vi "Swerve Offset.vi"() -> ()   [LabVIEW 2017]
uses:
  Robot Global Data.vi
  <vilib>/Rock Robotics/WPI/ThirdParty/Phoenix-LabVIEW/Motor Controller/Get/CTRE_Phoenix_MotorController_GetPulseWidthAll.vi
panel:
  in  "Z":dbl(slide) scale=-1.0..1.0
  in  "X":dbl(slide) scale=-1.0..1.0
  in  "Y":dbl(slide)=0.2448979591836733 scale=-1.0..1.0
  in  "Offsets":dbl[](array[knob])=[-0.26448025674899267, -0.387138341978177, -0.11650266473879117, -0.12073098447218328] scale=-0.5..0.5
  in  "Change":bool
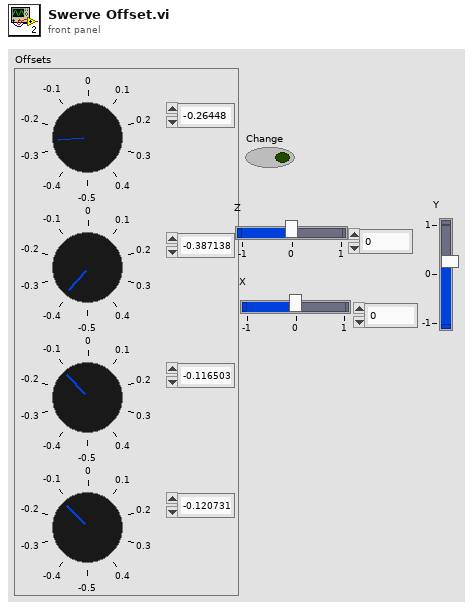
[diagram p1: front panel]
types:
  T1 = typedef "WPI_MotorControlDeviceRef.ctl" = cluster{"DeviceStatus":errorcluster, "Type":T2, "PWM":cluster{"PWM Channel":T3, "DeadBand":T4}, "CAN":cluster{"Device Number":u8, "SetOutput VI Ref":variant, "GetOutput VI Ref":variant, "Enable VI Ref":variant, "Disable VI Ref":variant, "Data":variant}, "Invert":bool, "DIO PWM":cluster{"PWM \"Enable\" Channel":T3, "DIOChannel":T5, "PWM Rate":dbl}}
  T2 = typedef "WPI_MotorControlType.ctl" = enum16{"PWM", "CAN", "DIO PWM"}
  T3 = typedef "FPGA_DIOPWMChannel.ctl" = enum8{"PWM 0", "PWM 1", "PWM 2", "PWM 3", "PWM 4", "PWM 5", "PWM 6", "PWM 7", "PWM 8", "PWM 9", "PWM MXP 0", "PWM MXP 1", "PWM MXP 2", "PWM MXP 3", "PWM MXP 4", "PWM MXP 5", "PWM MXP 6", "PWM MXP 7", "PWM MXP 8", "PWM MXP 9", "Invalid"}
  T4 = typedef "WPI_PWMDeadband.ctl" = cluster{"Name":string, "maxPositivePwm":i32, "minPositivePwm":i32, "centerPwm":i32, "maxNegativePwm":i32, "minNegativePwm":i32, "angularRange":u16}
  T5 = typedef "FPGA_DIOChannel.ctl" = enum8{"DIO 0", "DIO 1", "DIO 2", "DIO 3", "DIO 4", "DIO 5", "DIO 6", "DIO 7", "DIO 8", "DIO 9", "DIO MXP 0", "DIO MXP 1", "DIO MXP 2", "DIO MXP 3", "DIO MXP 4", "DIO MXP 5", "DIO MXP 6", "DIO MXP 7", "DIO MXP 8", "DIO MXP 9", "DIO MXP 10", "DIO MXP 11", "DIO MXP 12", "DIO MXP 13", "DIO MXP 14", "DIO MXP 15", "SPI Port CS1", "SPI Port CS2", "SPI Port CS3", "SPI Port MISO", "SPI Port MOSI", "Invalid"}
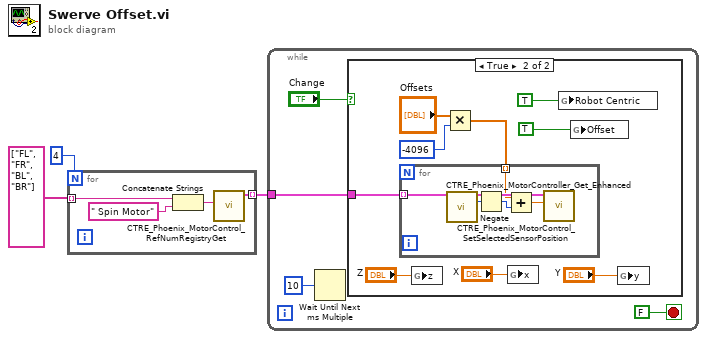
[diagram p0: block diagram]
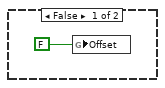
[diagram p2: hidden frame]
diagram:
  n1 = for {
    N: 4 -> [_]
    tunnel: string[] ["FL", "FR", "BL", "BR"] -> [w5] mode=indexing
    tunnel: [w4] -> w1 mode=indexing
    n2 = Concatenate Strings(w5, " Spin Motor" ("refnum name")) -> (w7:string)
    n3 = call <vilib>:"CTRE_Phoenix_MotorControl_RefNumRegistryGet.vi"("refnum name"=w7) -> ("PhoenixMotorControlDevRef"=w4:T1)  [unwired: 9 in, 1 out]
  }
  n4 = while {
    tunnel: w1 -> [w8]
    stop <- FALSE stop-if-true
    n5 = Wait Until Next ms Multiple(millisecond multiple=u32 10) -> ()  [unwired: 1 out]
    n6 = case shown="True" "Change" {
      tunnel: w8 -> [_ w20]
      frame False {
        n7 = global write "Robot Global Data.vi" "Offset"(FALSE) -> ()
      }
      frame True {
        n8 = global write "Robot Global Data.vi" "z"("Z") -> ()
        n9 = Multiply(x="Offsets", y=-4096) -> (x*y=w14:dbl[])
        n10 = for {
          tunnel: w20 -> [w26] mode=indexing
          tunnel: w14 -> [w24] mode=indexing
          n11 = call-poly <vilib>:"CTRE_Phoenix_MotorController_Get_Enhanced.vi"("PhoenixMotorControlDevRef"=w26) -> ("PhoenixMotorControlDevRef"=w27:T1, "Pulse Width Position"=w25:i32)  [unwired: 9 in, 4 out]
          n12 = Negate(x=w25) -> (-x=w22:i32)
          n13 = Add(x=w24, y=w22) -> (x+y=w23:dbl)
          n14 = call <vilib>:"CTRE_Phoenix_MotorControl_SetSelectedSensorPosition.vi"("New Sensor Position"=w23, "PhoenixMotorControlDevRef"=w27) -> ()  [unwired: 8 in, 2 out]
        }
        n15 = global write "Robot Global Data.vi" "x"("X") -> ()
        n16 = global write "Robot Global Data.vi" "Robot Centric"(TRUE ("Robot Centric")) -> ()
        n17 = global write "Robot Global Data.vi" "Offset"(TRUE) -> ()
        n18 = global write "Robot Global Data.vi" "y"("Y") -> ()
      }
    }
  }
